vi "testFact.vi"() -> (0 "error out":errorcluster)   [LabVIEW 2019, in "TestSuiteTest.lvlib" / "Create.lvlib"]
uses:
  Create.lvlib
  TestSuite/TestSuite.lvclass
  Assertion/Assertion.lvlib
  TestSuiteTestSupport/TestSuiteTestSupport.lvlib
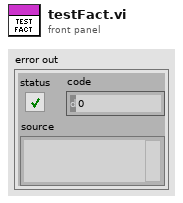
[diagram p1: front panel]
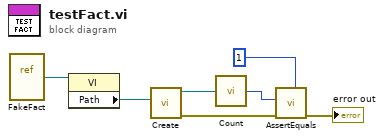
[diagram p0: block diagram]
diagram:
  n1 = vi-ref "FakeFact.vi"() -> (w3:refnum<vi>)
  n2 = property class="VI"(reference=w3) -> ("Path"=w2:path)  [unwired: 1 in, 2 out]
  n3 = call "Create.vi"("Path"=w2) -> ("error out"=w5:errorcluster, "TestSuite"=w7:refnum<class "TestSuite.lvclass">)  [unwired: 9 in]
  n4 = call "Count.vi"("TestSuite In"=w7) -> ("Count"=w6:i32)
  n5 = call "AssertEquals.vi"("Expected"=1 ("Count"), "error in (no error)"=w5, "Actual"=w6) -> ("error out"=→"error out":errorcluster)  [unwired: 8 in]
